vi "Create.vi"(8 "error in (no error)":errorcluster, 9 "Bid":u64, 10 "Input":string) -> (0 "error out":errorcluster, 3 "Hand":refnum<class "Hand.lvclass">)   [LabVIEW 2020, in "Hand.lvclass"]
uses:
  Hand.lvclass
  Hand.lvclass/Hand.ctl
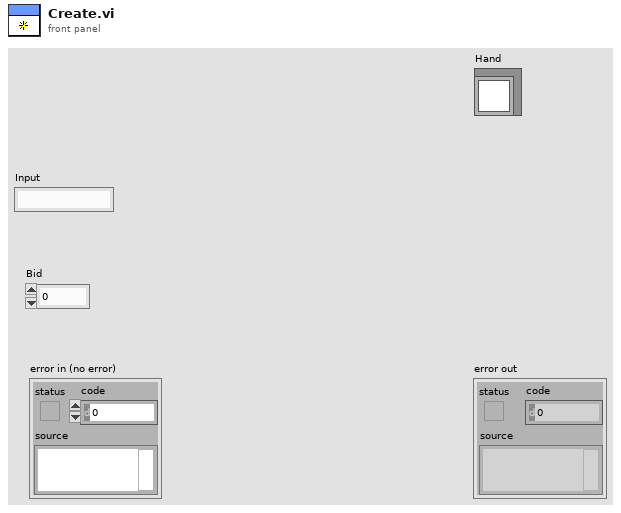
[diagram p1: front panel]
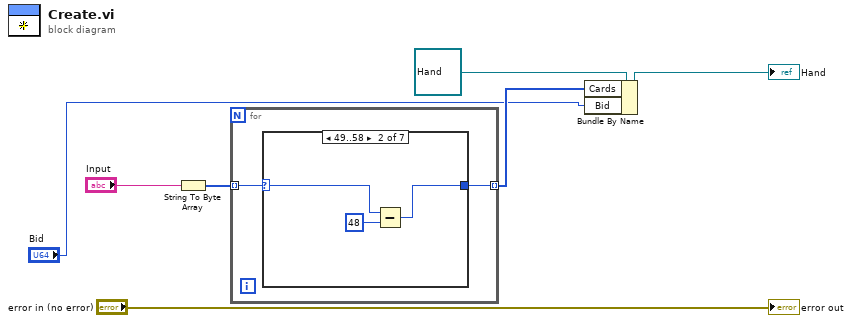
[diagram p0: block diagram]
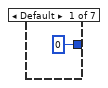
[diagram p2: hidden frame]
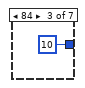
[diagram p3: hidden frame]
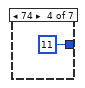
[diagram p4: hidden frame]
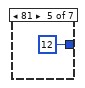
[diagram p5: hidden frame]
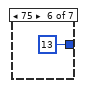
[diagram p6: hidden frame]
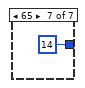
[diagram p7: hidden frame]
diagram:
  n1 = String To Byte Array(string="Input") -> (unsigned byte array=w4:u8[])
  n2 = for {
    tunnel: w4 -> [w9] mode=indexing
    tunnel: [w8] -> w2 mode=indexing
    n3 = case shown="49..58" w9 {
      selector: w9 -> [_ w12 _ _ _ _ _]
      tunnel: [u8 0 w11 u8 10 u8 11 u8 12 u8 13 u8 14] -> w8
      frame Default {
      }
      frame 49..58 {
        n4 = Subtract(x=w12, y=u8 48) -> (x-y=w11:u8)
      }
      frame 84 {
      }
      frame 74 {
      }
      frame 81 {
      }
      frame 75 {
      }
      frame 65 {
      }
    }
  }
  n5 = Bundle By Name(cluster=refnum<class "Hand.lvclass"> refnum ("Hand"), "Cards"=w2, "Bid"="Bid") -> (→"Hand":refnum<class "Hand.lvclass">)
  "error out" <- "error in (no error)"
